vi "testTransceiverTest.vi"(8 "error in (no error)":errorcluster, 11 "TestCase in":refnum<class "DSFPluginTestCase.lvclass">) -> (0 "error out":errorcluster, 3 "TestCase out":refnum<class "DSFPluginTestCase.lvclass">)   [LabVIEW 2017, in "DSFPluginTestCase.lvclass"]
uses:
  DSFPluginTestCase.lvclass
  <vilib>/ErrorRing/Error Ring.xnode
  <vilib>/addons/_JKI Toolkits/VI Tester/TestCase.llb/TestCase.lvclass
  C:/Program Files (x86)/National Instruments/LabVIEW 2017/vi.lib/addons/_JKI Toolkits/VI Tester/TestCase.llb/TestCase.lvclass
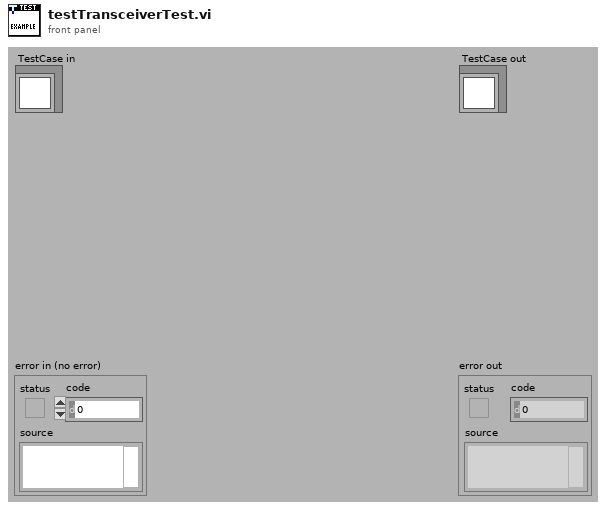
[diagram p1: front panel]
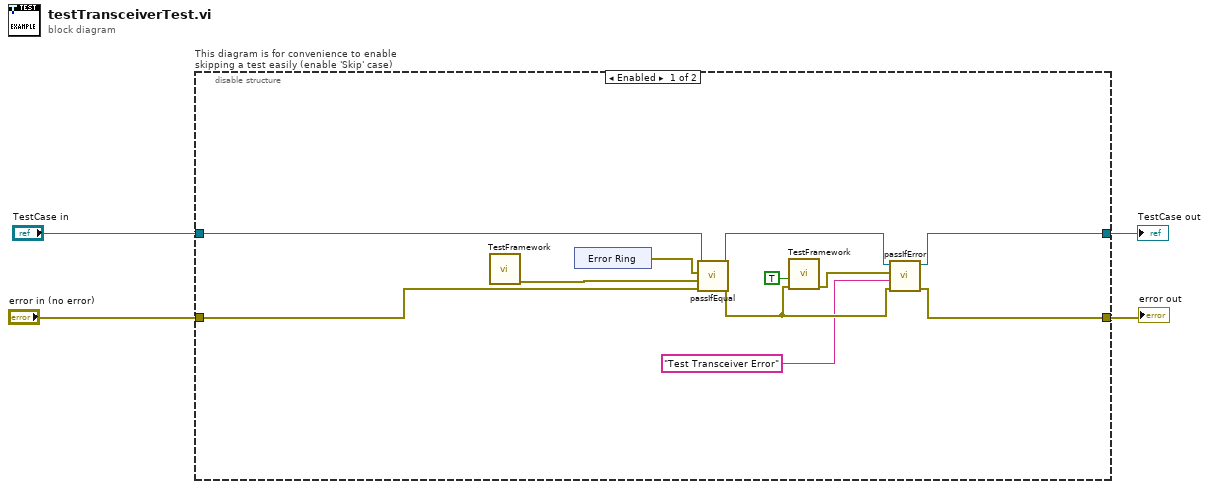
[diagram p0: block diagram]
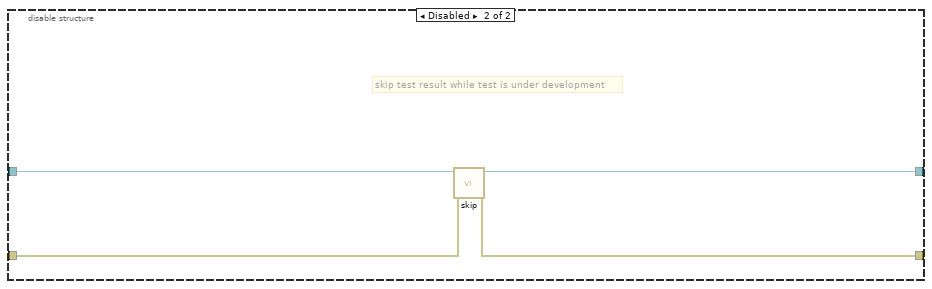
[diagram p2: hidden frame]
diagram:
  n1 = disable-structure "This diagram is for convenience to enable skipping a test easily (enable 'Skip' case)" shown="Enabled" {
    disable-tunnel: "TestCase in" -> [w15 w20]
    disable-tunnel: [w6 w18] -> w1
    disable-tunnel: [w8 w19] -> w3
    disable-tunnel: "error in (no error)" -> [w12 w17]
    frame Enabled {
      n2 = call "TestFramework.vi"() -> ("error out"=w14:errorcluster)  [unwired: 10 in, 1 out]
      n3 = xnode "Error Ring"() -> ("error out"=w13:errorcluster)
      n4 = call-dynamic "passIfEqual.vi"("error in (no error)"=w12, "y"=w14, "x"=w13, "TestCase in"=w15) -> ("error out"=w10:errorcluster, "TestCase out"=w7:refnum<class "DSFPluginTestCase.lvclass">)  [unwired: 6 in]
      n5 = call "TestFramework.vi"("error in (no error)"=w10, "Simulate Error?"=TRUE) -> ("error out"=w9:errorcluster)  [unwired: 8 in, 1 out]
      n6 = call-dynamic "passIfError.vi"("error in (no error)"=w10, "task (\"\")"="Test Transceiver Error" ("task (\"\")"), "error"=w9, "TestCase in"=w7) -> ("error out"=w8:errorcluster, "TestCase out"=w6:refnum<class "DSFPluginTestCase.lvclass">)  [unwired: 6 in]
    }
    frame Disabled {
      # "skip test result while test is under development"
      n7 = call <vilib>:"skip.vi"("error in (no error)"=w17, "TestCase in"=w20) -> ("error out"=w19:errorcluster, "TestCase out"=w18:refnum<class "DSFPluginTestCase.lvclass">)  [unwired: 8 in]
    }
  }
  "error out" <- w3
  "TestCase out" <- w1
